vi "Set Self Enqueuer.vi"(8 "error in (no error)":errorcluster, 10 "Self Enqueuer":refnum<class "Message Enqueuer.lvclass">, 11 "Add Form to Database Button in":refnum<class "Add Form to Database Button.lvclass">) -> (0 "error out":errorcluster, 3 "Add Form to Database Button out":refnum<class "Add Form to Database Button.lvclass">)   [LabVIEW 2020]
uses:
  Add Form to Database Button.lvclass
  <vilib>/ActorFramework/Message Enqueuer/Message Enqueuer.lvclass
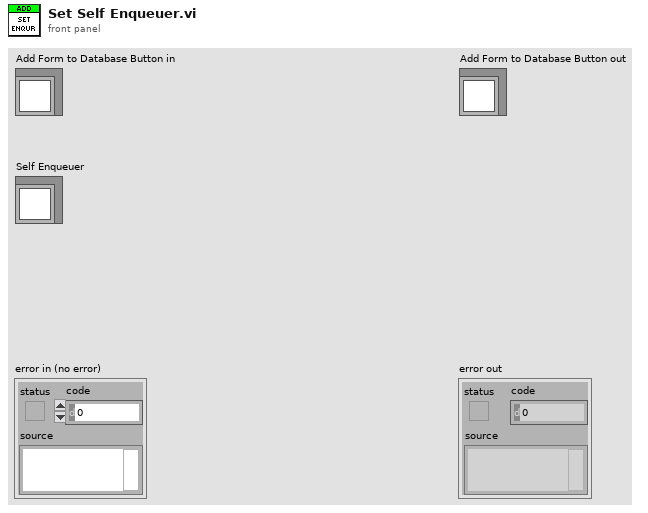
[diagram p1: front panel]
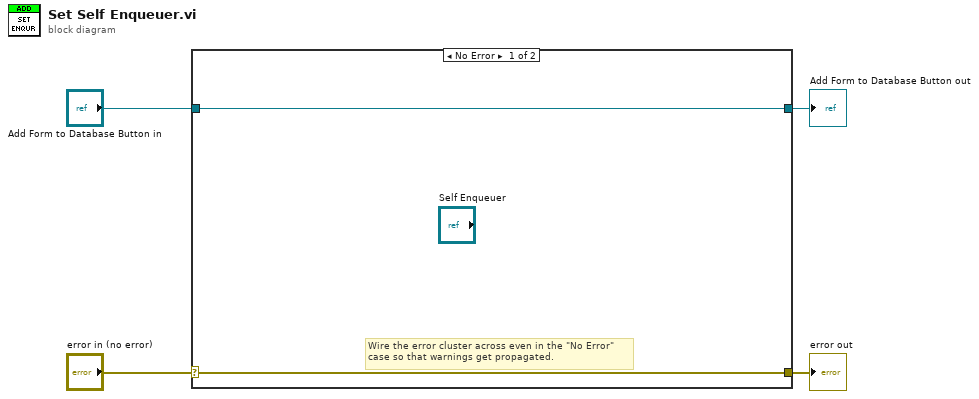
[diagram p0: block diagram]
diagram:
  n1 = case shown="No Error" "error in (no error)" {
    selector: "error in (no error)" -> [w5 w8]
    tunnel: [w5 w8] -> w3
    tunnel: [w6 w7] -> w1
    tunnel: "Add Form to Database Button in" -> [w6 w7]
    frame No Error {
      # "Wire the error cluster across even in the \"No Error\"\ncase so that warnings get propagated."
    }
    frame Error {
    }
  }
  "error out" <- w3
  "Add Form to Database Button out" <- w1
